vi "Calc time of measurement new.vi"(1 "Number of Power Line Cycles(50Hz)":dbl=50.0, 2 "2182 -A Params":T1={"Auto Range?"=FALSE, "Man / Selected\n       Range"=enum."10mV", "Enable Digital\n       Filter?"=FALSE, "Filter Type"=enum."Movin", "Filter Count"=1, "      Filter\nWindow (%)"=0.01, "Enable Analog\n       Filter?"=FALSE, "NPLCs"=5} {"NPLCs" min=1 max=10; "Filter\nWindow (%)" min=0.01 max=10.0 step=0.01 format="%.2f"; "Filter Count" min=1 max=100}) -> (0 "Time of one measurement":dbl=7100.0)   [LabVIEW 2013, in "Keithly user program.lvlib"]
uses:
  Keithly user program.lvlib
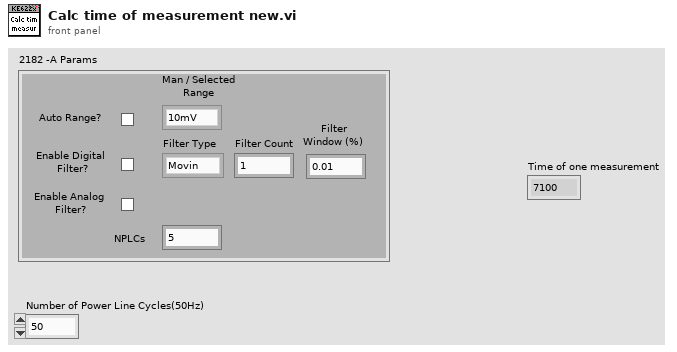
[diagram p1: front panel]
types:
  T1 = cluster{"Auto Range?":bool, "Man / Selected\n       Range":enum16{"10mV", "100mV", "1V", "10V", "100V"}, "Enable Digital\n       Filter?":bool, "Filter Type":enum16{"Movin", "Repeat"}, "Filter Count":u32, "      Filter\nWindow (%)":dbl, "Enable Analog\n       Filter?":bool, "NPLCs":u32}
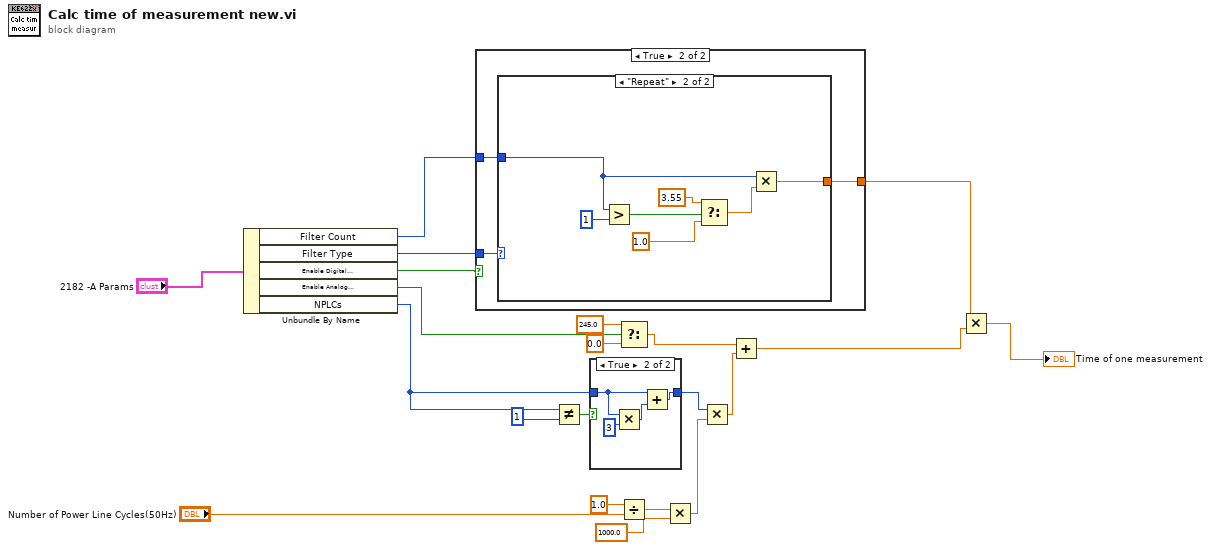
[diagram p0: block diagram]
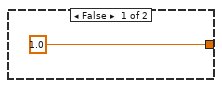
[diagram p2: hidden frame]
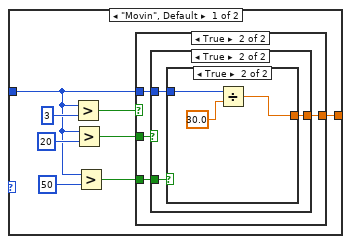
[diagram p3: hidden frame]
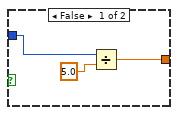
[diagram p5: hidden frame]
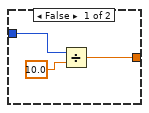
[diagram p6: hidden frame]
diagram:
  n1 = Unbundle By Name("2182 -A Params") -> ("Filter Count"=w1:u32, "Filter Type"=w3:enum16{"Movin", "Repeat"}, "Enable Digital\n       Filter?"=w4:bool, "Enable Analog\n       Filter?"=w15:bool, "NPLCs"=w13:u32)
  n2 = case shown="True" w4 {
    tunnel: w3 -> [_ w25]
    tunnel: [1.0 ("s? t:f") w23] -> w2
    tunnel: w1 -> [_ w24]
    frame False {
    }
    frame True {
      n3 = case shown="\"Repeat\"" w25 {
        tunnel: w24 -> [w27 w55]
        tunnel: [w26 w53] -> w23
        frame "Movin", Default {
          n4 = Greater?(x=w27, y=u32 3) -> (0:w30:bool)
          n5 = Greater?(x=w27, y=u32 20) -> (0:w29:bool)
          n6 = Greater?(x=w27, y=u32 50) -> (0:w28:bool)
          n7 = case shown="True" w30 {
            tunnel: w29 -> [_ w38]
            tunnel: w28 -> [_ w37]
            tunnel: w27 -> [w34 w36]
            tunnel: [w34 w35] -> w26
            frame False {
            }
            frame True {
              n8 = case shown="True" w38 {
                tunnel: w37 -> [_ w44]
                tunnel: w36 -> [w40 w43]
                tunnel: [w39 w42] -> w35
                frame False {
                  n9 = Divide(x=w40, y=5.0 ("f")) -> (x/y=w39:dbl)
                }
                frame True {
                  n10 = case shown="True" w44 {
                    tunnel: w43 -> [w47 w50]
                    tunnel: [w46 w48] -> w42
                    frame False {
                      n11 = Divide(x=w47, y=10.0 ("f")) -> (x/y=w46:dbl)
                    }
                    frame True {
                      n12 = Divide(x=w50, y=30.0 ("f")) -> (x/y=w48:dbl)
                    }
                  }
                }
              }
            }
          }
        }
        frame "Repeat" {
          n13 = Greater?(x=w55, y=u32 1) -> (0:w56:bool)
          n14 = Select(t=3.55, s=w56, f=1.0) -> (s? t:f=w54:dbl)
          n15 = Multiply(x=w55, y=w54) -> (x*y=w53:dbl)
        }
      }
    }
  }
  n16 = Not Equal?(x=w13, y=u32 1) -> (x != y?=w12:bool)
  n17 = case shown="True" w12 {
    tunnel: w13 -> [w58 w60]
    tunnel: [w58 w62] -> w14
    frame False {
    }
    frame True {
      n18 = Multiply(x=w60, y=u32 3) -> (x*y=w61:u32)
      n19 = Add(x=w60, y=w61) -> (x+y=w62:u32)
    }
  }
  n20 = Select(t=245.0, s=w15, f=0.0) -> (s? t:f=w18:dbl)
  n21 = Divide(x=1.0, y="Number of Power Line Cycles(50Hz)") -> (x/y=w8:dbl)
  n22 = Multiply(x=w8, y=1000.0) -> (x*y=w10:dbl)
  n23 = Multiply(x=w14, y=w10) -> (x*y=w19:dbl)
  n24 = Add(x=w18, y=w19) -> (x+y=w20:dbl)
  n25 = Multiply(x=w2, y=w20) -> (x*y=→"Time of one measurement":dbl)
